vi "nirvififoPalette_MergeVI.vi"   [LabVIEW 2017]
doc: "Invokes a FIFO method on an FPGA VI. You can invoke some or all of the following methods on FPGA FIFOs. The methods you can choose from depend on the FIFO you specify. \n\nYou must specify a FIFO before you specify a method.\n\nClear\n\nRead\n\nWrite\n\nDisable\n\nEnable\n\nFlush and Disable\n\nGet Stream State\n\nGet Number of Elements to Write\n\nGet Number of Elements to Read"
uses:
  <vilib>/rvi/DataTransferAndStorage/Container/XNode/niFpgaContainer.xnode
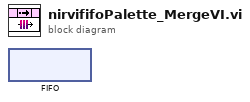
[diagram p0: block diagram]
diagram:
  n1 = xnode "FIFO"() -> ()  [unwired: 1 in, 1 out]
